vi "getChannelName.vi"(8 "error in (no error)":errorcluster, 11 "ScriptEvent in":refnum<class "ScriptEvent.lvclass">) -> (0 "error out":errorcluster, 2 "channel_name":string, 3 "ScriptEvent out":refnum<class "ScriptEvent.lvclass">)   [LabVIEW 2011, in "Tools.lvlib" / "Scripting.lvlib" / "ScriptEvent.lvclass"]
uses:
  ScriptEvent.lvclass
  ScriptEvent.lvclass/ScriptEvent.ctl
  DatabaseHelpers/Database Objects/Channel/Channel.lvclass
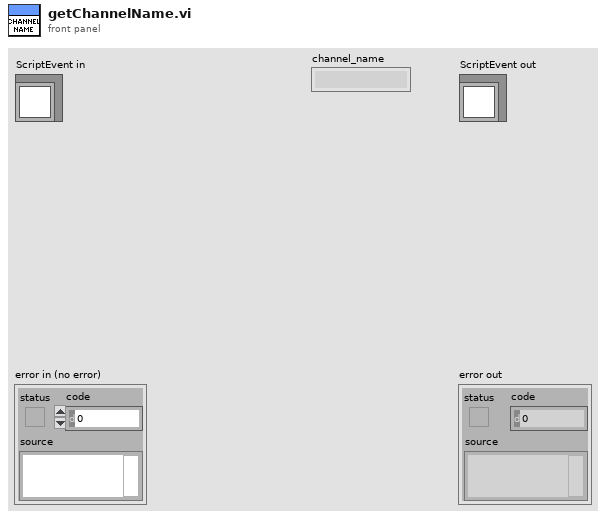
[diagram p1: front panel]
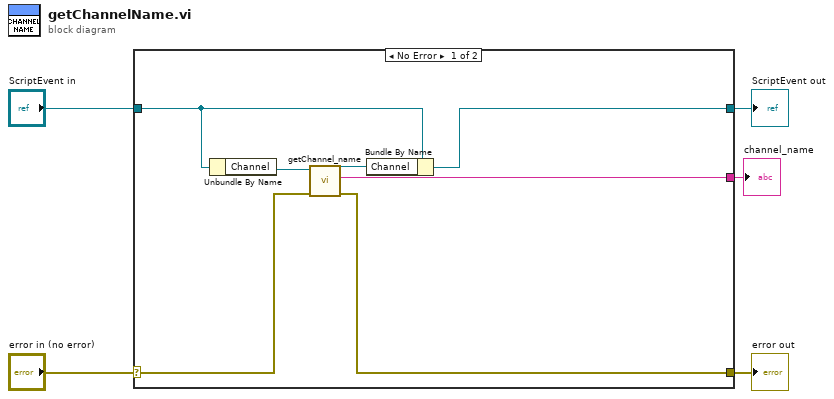
[diagram p0: block diagram]
diagram:
  n1 = case shown="No Error" "error in (no error)" {
    selector: "error in (no error)" -> [w8 w14]
    tunnel: [w7 w14] -> w4
    tunnel: [w9 w13] -> w2
    tunnel: "ScriptEvent in" -> [w10 w13]
    tunnel: [w6 _] -> w1
    frame No Error {
      n2 = Unbundle By Name(w10) -> ("Channel"=w12:refnum<class "Channel.lvclass">)
      n3 = call "getChannel_name.vi"("error in (no error)"=w8, "Channel.lvclass in"=w12) -> ("error out"=w7:errorcluster, "channel_name"=w6:string, "Channel.lvclass out"=w11:refnum<class "Channel.lvclass">)  [unwired: 7 in]
      n4 = Bundle By Name(cluster=w10, "Channel"=w11) -> (w9:refnum<class "ScriptEvent.lvclass">)
    }
    frame Error {
    }
  }
  "error out" <- w4
  "ScriptEvent out" <- w2
  "channel_name" <- w1
